vi "Rodolfo glitch test.vi"() -> ()   [LabVIEW 2012]
panel:
  out "Corrected Av":dbl
  out "Corrected Rv":dbl
  out "Final Av":dbl
  out "Final Rv":dbl
  in  "iterations calibration acq":u32
  in  "Fine Retraction":dbl
  in  "Fine Approach":dbl
  in  "Final":i32=-5529
  in  "Initial":i32=-5725
  in  "Calculation Ready":bool=TRUE
  out "Stage-calibration":i16=1
  in  "Data for Velocity Calculation":bool
  in  "Step-length-pzt":i16=50
  in  "Calibration Wait Time (ms)":u32=3000
  in  "Period Calibration Acq":u32=2000
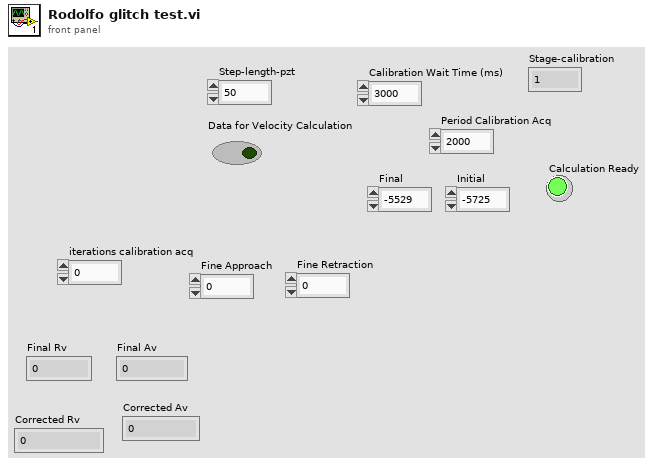
[diagram p1: front panel]
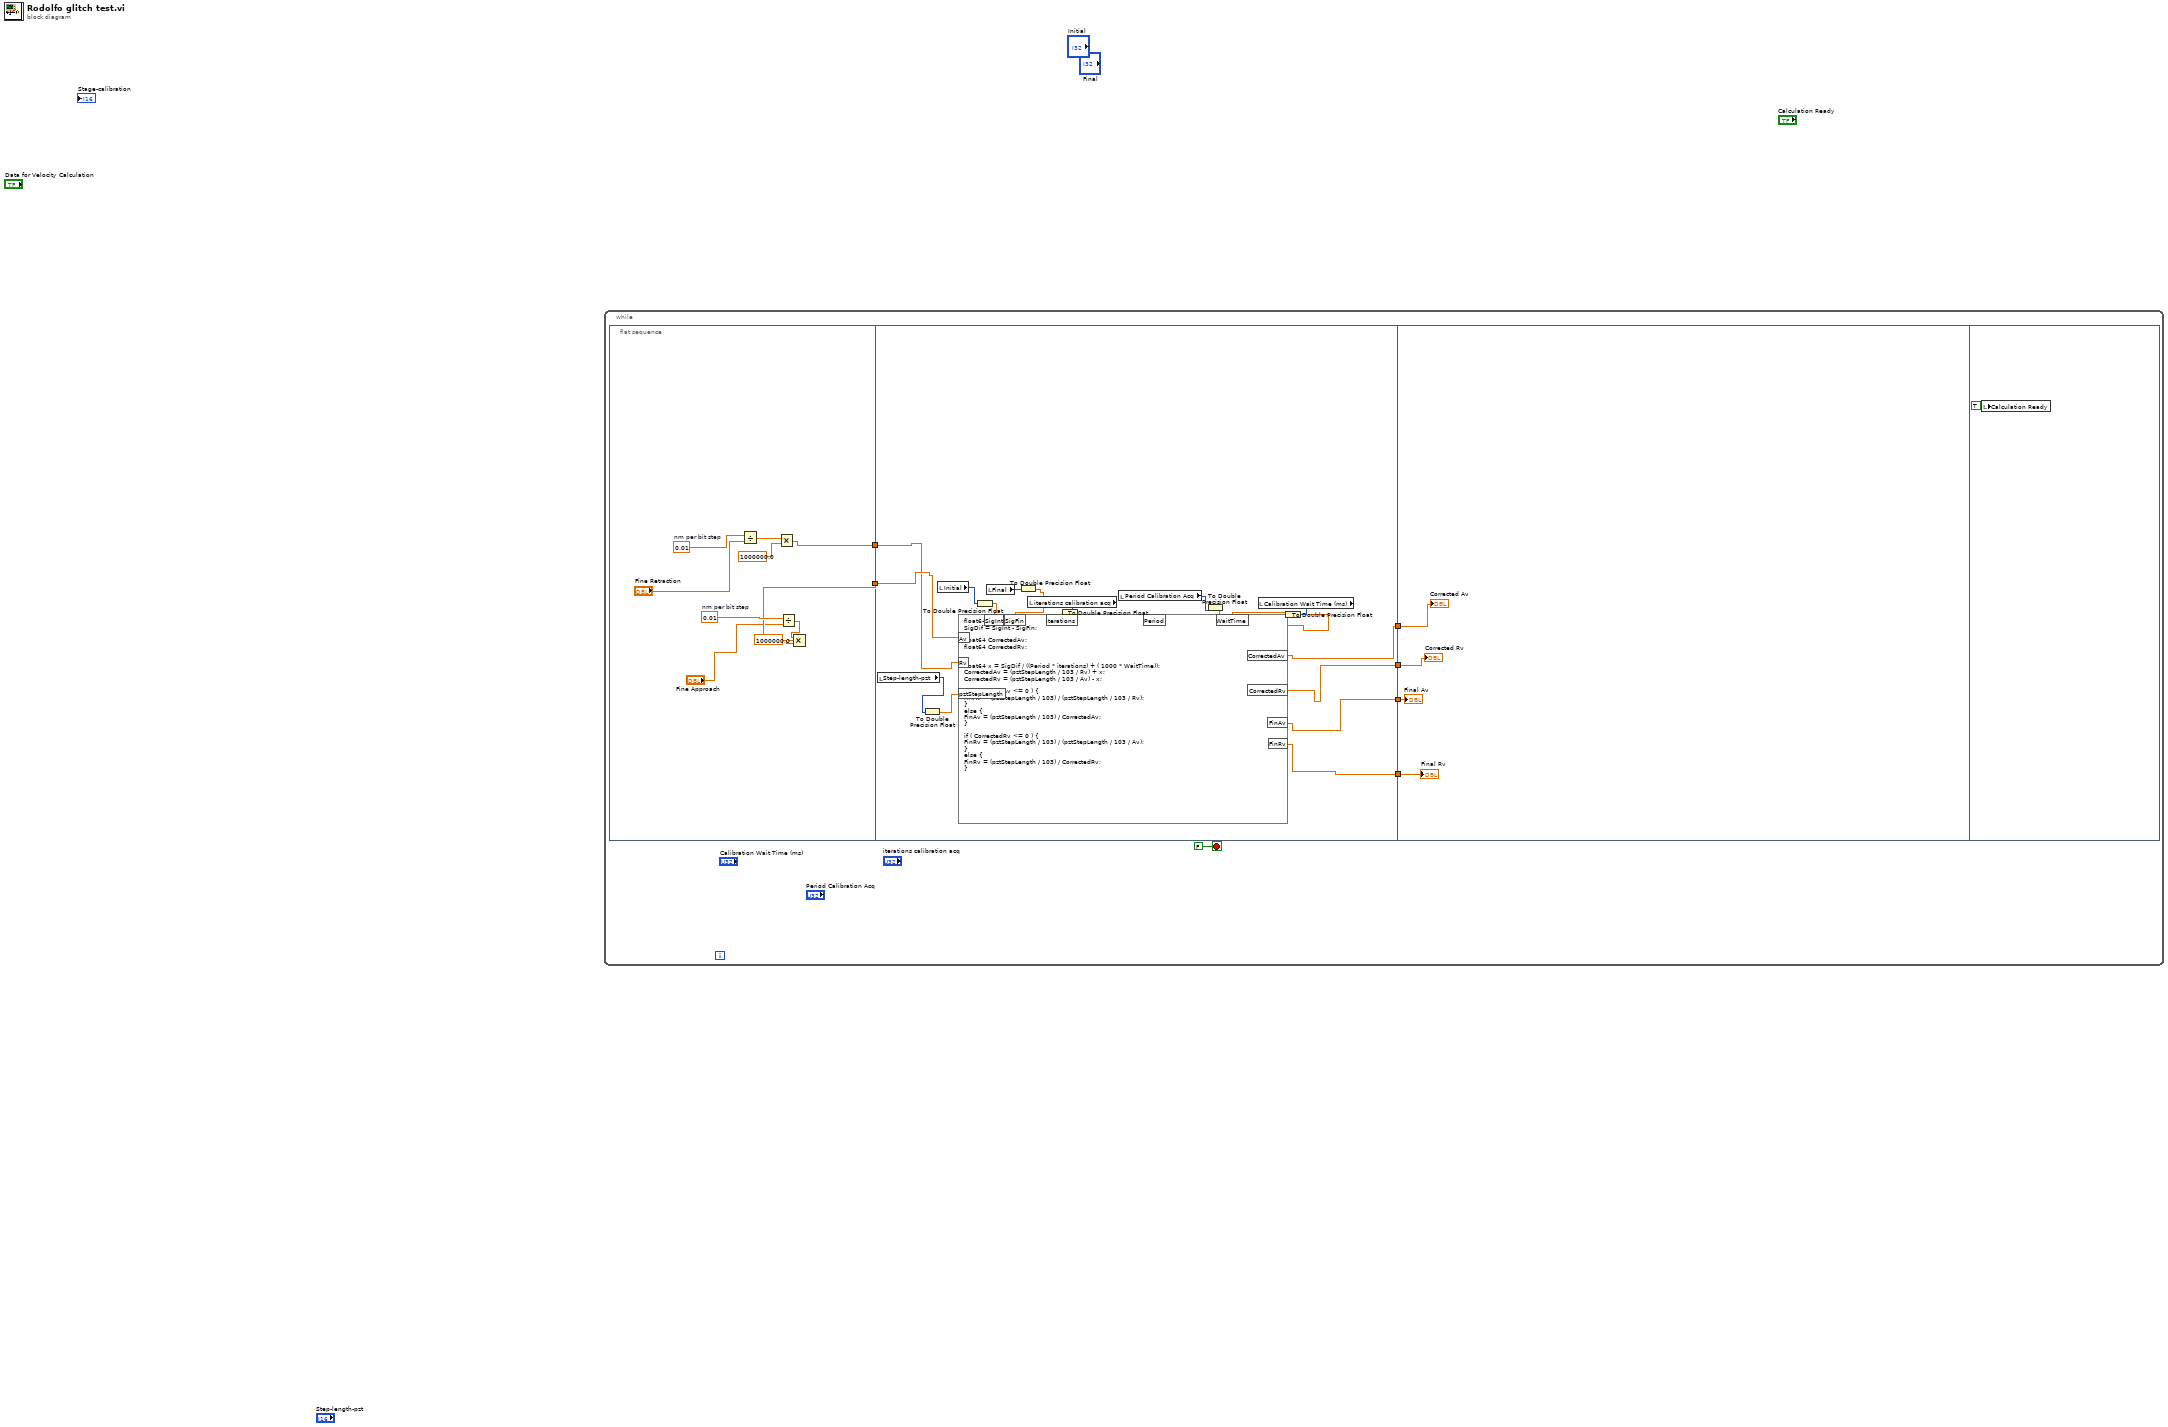
[diagram p0: block diagram]
diagram:
  n1 = while {
    stop <- FALSE stop-if-true
    n2 = flat-sequence {
      tunnel: [w11] -> w6
      tunnel: [w10] -> w5
      tunnel: w6 -> [w22]
      tunnel: w5 -> [w35]
      tunnel: [w21] -> w4
      tunnel: [w20] -> w3
      tunnel: [w19] -> w2
      tunnel: [w18] -> w1
      tunnel: w4 -> [w39]
      tunnel: w3 -> [w38]
      tunnel: w2 -> [w37]
      tunnel: w1 -> [w36]
      frame #0 {
        w14 = 0.01  # nm per bit step
        w17 = 0.01  # nm per bit step
        n3 = Divide(x=w14, y="Fine Retraction") -> (x/y=w13:dbl)
        n4 = Multiply(x=w13, y=1000000.0) -> (x*y=w11:dbl)
        n5 = Divide(x=w17, y="Fine Approach") -> (x/y=w16:dbl)
        n6 = Multiply(x=w16, y=1000000.0) -> (x*y=w10:dbl)
      }
      frame #1 {
        n7 = local read "Step-length-pzt"() -> (w24:i16)
        n8 = To Double Precision Float(number=w24) -> (double precision float=w23:dbl)
        n9 = local read "Initial"() -> (w34:i32)
        n10 = To Double Precision Float(number=w34) -> (double precision float=w33:dbl)
        n11 = local read "Final"() -> (w32:i32)
        n12 = To Double Precision Float(number=w32) -> (double precision float=w31:dbl)
        n13 = local read "iterations calibration acq"() -> (w30:u32)
        n14 = To Double Precision Float(number=w30) -> (double precision float=w29:dbl)
        n15 = local read "Period Calibration Acq"() -> (w28:u32)
        n16 = To Double Precision Float(number=w28) -> (double precision float=w27:dbl)
        n17 = local read "Calibration Wait Time (ms)"() -> (w26:u32)
        n18 = To Double Precision Float(number=w26) -> (double precision float=w25:dbl)
        n19 = formula code="float64 SigDif;\nSigDif = SigInt - SigFin;\n\nfloat64 CorrectedAv;\nfloat64 CorrectedRv;\n\n\nfloat64 x = SigDif / ((Period * iterations) + ( 1000 * WaitTime));\nCorrectedAv = (pztStepLength / 103 / Rv) + x;\nCorrectedRv = (pztStepLength / 103 / Av) - x; \n\nif ( CorrectedAv <= 0 ) {\nFinAv = (pztStepLength / 103) / (pztStepLength / 103 / Rv); \n}\nelse {\nFinAv = (pztStepLength / 103) / CorrectedAv;\n}\n\nif ( CorrectedRv <= 0 ) {\nFinRv = (pztStepLength / 103) / (pztStepLength / 103 / Av);\n}\nelse {\nFinRv = (pztStepLength / 103) / CorrectedRv;\n}"("Period"=w27, "Av"=w35, "Rv"=w22, "SigInt"=w33, "SigFin"=w31, "iterations"=w29, "WaitTime"=w25, "pztStepLength"=w23) -> ("CorrectedAv"=w18:dbl, "CorrectedRv"=w19:dbl, "FinAv"=w20:dbl, "FinRv"=w21:dbl)
      }
      frame #2 {
        "Corrected Av" <- w36
        "Corrected Rv" <- w37
        "Final Av" <- w38
        "Final Rv" <- w39
      }
      frame #3 {
        n20 = local write "Calculation Ready"(TRUE ("Calculation Ready")) -> ()
      }
    }
  }
